vi "TENMA 72-2710 general control.vi"(6 "Value to set":sgl, 7 "Command":T1="*IDN?", 8 "Port":refnum<visa-resource-name>) -> (0 "Output enabled":bool, 1 "error out":errorcluster, 2 "CV mode":bool, 3 "Returned string":string, 5 "Returned value":sgl=nan format="%_4g")   [LabVIEW 2022 SP3]
uses:
  ctls/TENMA 72-2xxx commands.ctl
  <vilib>/Instr/_visa.llb/VISA Open Access Mode.ctl
panel:
  # "PN 13/04/18"
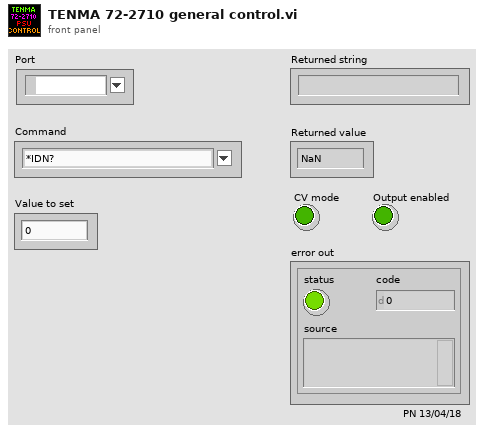
[diagram p1: front panel]
types:
  T1 = typedef "TENMA 72-2xxx commands.ctl" = string
  T2 = typedef "VISA Open Access Mode.ctl" = u32
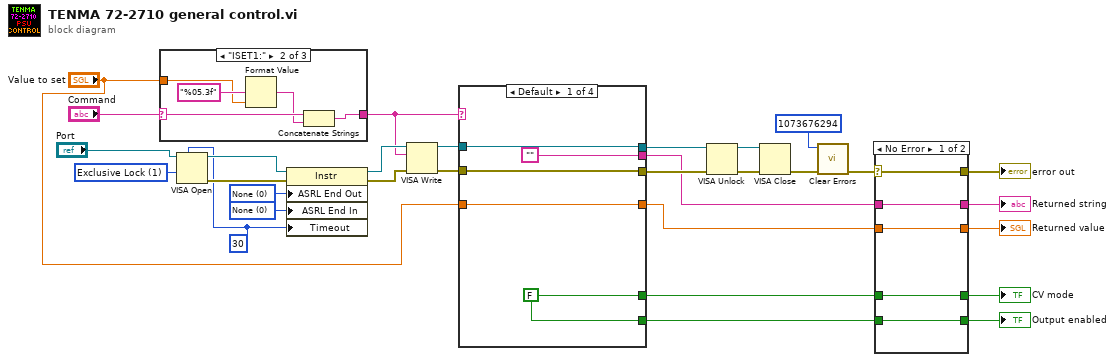
[diagram p0: block diagram]
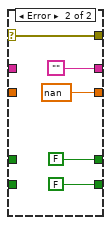
[diagram p2: hidden frame]
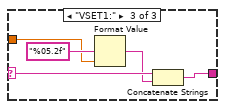
[diagram p4: hidden frame]
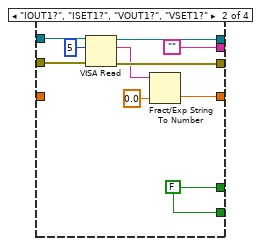
[diagram p5: hidden frame]
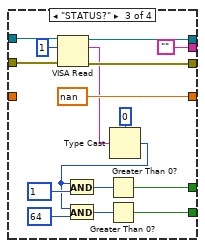
[diagram p6: hidden frame]
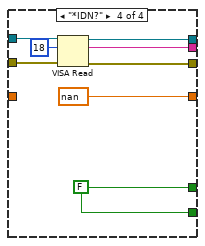
[diagram p7: hidden frame]
diagram:
  w1 = u32 30 ("General Settings:Timeout Value")
  w19 = u16 0 items=["None", "Last Bit", "TermChar"] ("Serial Settings:End Mode for Reads")
  w20 = u16 0 items=["None", "Last Bit", "TermChar", "Break"] ("Serial Settings:End Mode for Writes")
  w30 = T2 1 items=["VISA Defaults"=0, "Exclusive Lock"=1, "Load Configured Settings"=4] ("Access Mode")
  n1 = case shown="\"ISET1:\"" "Command" {
    selector: "Command" -> [w31 w36 w41]
    tunnel: [w31 w35 w40] -> w13
    tunnel: "Value to set" -> [_ w33 w38]
    frame Default {
    }
    frame "ISET1:" {
      n2 = Format Value(format string="%05.3f", value (0)=w33) -> (output string=w32:string)  [unwired: 1 in]
      n3 = Concatenate Strings(w36, w32) -> (w35:string)
    }
    frame "VSET1:" {
      n4 = Format Value(format string="%05.2f", value (0)=w38) -> (output string=w37:string)  [unwired: 1 in]
      n5 = Concatenate Strings(w41, w37) -> (w40:string)
    }
  }
  n6 = VISA Open(timeout (0)=w1, access mode=w30, VISA resource name="Port") -> (VISA resource name=w24:refnum<visa-resource-name>, error out=w22:errorcluster)  [unwired: 2 in]
  n7 = property class="Instr"(reference=w24, error in=w22, "ASRL End Out"=w20, "ASRL End In"=w19, "Timeout"=w1) -> (reference out=w23:refnum<visa-resource-name>, error out=w21:errorcluster)
  n8 = VISA Write(VISA resource name=w23, write buffer=w13, error in (no error)=w21) -> (VISA resource name out=w16:refnum<visa-resource-name>, error out=w15:errorcluster)  [unwired: 1 out]
  n9 = case shown="Default" w13 {
    tunnel: [w45 w56 w72 w80] -> w26
    tunnel: [w46 w55 w71 w79] -> w25
    tunnel: ["" "" "" w78] -> w10
    tunnel: w16 -> [w46 w54 w70 w77]
    tunnel: w15 -> [w45 w53 w69 w76]
    tunnel: [w42 w49 sgl nan sgl nan] -> w9
    tunnel: [w43 w47 w61 w73] -> w8
    tunnel: [w43 w47 w57 w73] -> w7
    tunnel: "Value to set" -> [w42 _ _ _]
    frame Default {
      w43 = FALSE
    }
    frame "IOUT1?", "ISET1?", "VOUT1?", "VSET1?" {
      w47 = FALSE
      n10 = VISA Read(VISA resource name=w54, byte count=u32 5, error in (no error)=w53) -> (VISA resource name out=w55:refnum<visa-resource-name>, read buffer=w51:string, error out=w56:errorcluster)  [unwired: 1 out]
      n11 = Fract/Exp String To Number(string=w51, default (0 dbl)=sgl 0.0 ("default (0 DBL)")) -> (number=w49:sgl)  [unwired: 2 in, 1 out]
    }
    frame "STATUS?" {
      n12 = VISA Read(VISA resource name=w70, byte count=u32 1, error in (no error)=w69) -> (VISA resource name out=w71:refnum<visa-resource-name>, read buffer=w66:string, error out=w72:errorcluster)  [unwired: 1 out]
      n13 = Type Cast(type=u8 0, x=w66) -> (*(type *) &x=w60:u8)
      n14 = And(x=w60, y=u8 1) -> (x .and. y?=w62:u8)
      n15 = And(x=w60, y=u8 64) -> (x .and. y?=w58:u8)
      n16 = Greater Than 0?(x=w62) -> (x > 0?=w61:bool)
      n17 = Greater Than 0?(x=w58) -> (x > 0?=w57:bool)
    }
    frame "*IDN?" {
      w73 = FALSE
      n18 = VISA Read(VISA resource name=w77, byte count=u32 18, error in (no error)=w76) -> (VISA resource name out=w79:refnum<visa-resource-name>, read buffer=w78:string, error out=w80:errorcluster)  [unwired: 1 out]
    }
  }
  n19 = VISA Unlock(8:w26, 11:w25) -> (0:w29:errorcluster, 3:w28:refnum<visa-resource-name>)
  n20 = VISA Close(VISA resource name=w28, error in (no error)=w29) -> (error out=w27:errorcluster)
  n21 = call <vilib>:"Clear Errors.vi"("error in (no error)"=w27, "specific error code to clear (0: all)"=1073676294) -> ("error out"=w12:errorcluster)  [unwired: 4 in, 1 out]
  n22 = case shown="No Error" w12 {
    selector: w12 -> [w85 w90]
    tunnel: [w85 w90] -> w11
    tunnel: w10 -> [w84 _]
    tunnel: w9 -> [w83 _]
    tunnel: w8 -> [w82 _]
    tunnel: w7 -> [w81 _]
    tunnel: [w84 ""] -> w6
    tunnel: [w83 sgl nan] -> w5
    tunnel: [w82 FALSE] -> w4
    tunnel: [w81 FALSE] -> w3
    frame No Error {
    }
    frame Error {
    }
  }
  "error out" <- w11
  "Returned string" <- w6
  "Returned value" <- w5
  "CV mode" <- w4
  "Output enabled" <- w3
